vi "Init.vi"(4 "Gyro Full Scale Range":T8, 6 "Accel Full Scale Range":T9, 7 "I2C Channel":u8, 8 "error in (no error)":errorcluster, 9 "Clock Source":u8=1, 10 "Device Address":T10=104 items=["0x68"=104, "0x69"=105], 11 "LINX Resource":T1) -> (0 "error out":errorcluster, 3 "LINX Resource":T1)   [LabVIEW 2011, in "LVH-LINX.lvlib" / "MPU60X0.lvlib"]
doc: "Initializes the MPU-60X0 device setting the clock source and the full ranges for the accelerometer and gyro."
uses:
  <vilib>/LabVIEW Hacker/LINX/Public/Sensors/Accelerometer/MPU60X0/MPU60X0.lvlib
  <vilib>/LabVIEW Hacker/LINX/Public/Sensors/Accelerometer/MPU60X0/DeviceAddresses.ctl
  <vilib>/LabVIEW Hacker/LINX/Public/Sensors/Accelerometer/MPU60X0/AccelFullScaleRanges.ctl
  <vilib>/LabVIEW Hacker/LINX/Public/Sensors/Accelerometer/MPU60X0/GyroFullScaleRanges.ctl
  <vilib>/LabVIEW Hacker/LINX/Private/Type Defs/LINX Ref.ctl
  <vilib>/LabVIEW Hacker/LINX/Private/Type Defs/Platform.ctl
  <vilib>/LabVIEW Hacker/LINX/Private/Type Defs/Interface.ctl
  <vilib>/LabVIEW Hacker/LINX/Private/Device/Type Defs/LINX Device Config.ctl
  <vilib>/LabVIEW Hacker/LINX/Private/Device/Type Defs/TCP Config.ctl
  <vilib>/LabVIEW Hacker/LINX/Private/Type Defs/Device Family.ctl
  <vilib>/LabVIEW Hacker/LINX/Private/Device/Type Defs/Channels.ctl
  <vilib>/LabVIEW Hacker/LINX/LVH-LINX.lvlib
  <vilib>/LabVIEW Hacker/LINX/Private/Device/Device.lvlib
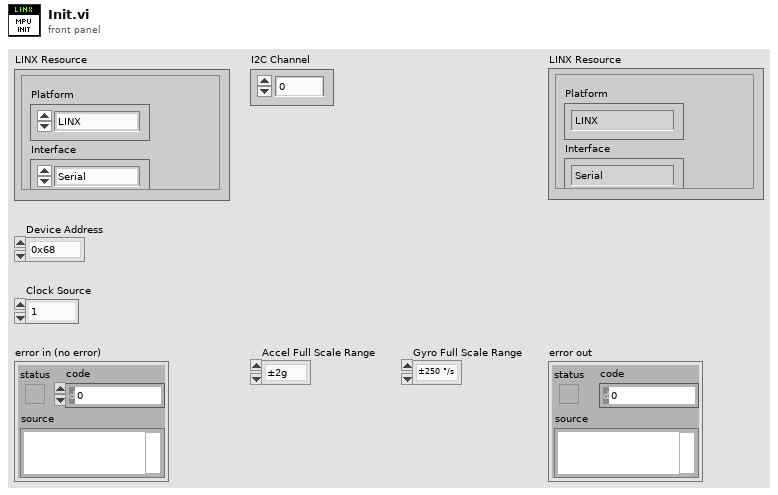
[diagram p1: front panel]
types:
  T1 = typedef "LVH-LINX.lvlib/LINX Ref.ctl" = cluster{"Platform":T2, "Interface":T3, "LINX Device Config":T4}
  T2 = typedef "LVH-LINX.lvlib/Platform.ctl" = enum16{"LINX", "myRIO"}
  T3 = typedef "LVH-LINX.lvlib/Interface.ctl" = enum16{"Serial", "TCP"}
  T4 = typedef "LVH-LINX.lvlib/Device.lvlib/LINX Device Config.ctl" = cluster{"Interface":T3, "COM Port":refnum<visa-resource-name>, "TCP Configuration":T5, "Device Family":T6, "Device ID":u8, "Device Name":string, "TCP Ref":refnum<k5>, "Channels":T7}
  T5 = typedef "LVH-LINX.lvlib/Device.lvlib/TCP Config.ctl" = cluster{"IP Address":string, "Port":u16}
  T6 = typedef "LVH-LINX.lvlib/Device Family.ctl" = enum8{"National Instruments", "Digilent", "Arduino"}
  T7 = typedef "LVH-LINX.lvlib/Channels.ctl" = cluster{"DI Channels":u8[], "DO Channels":u8[], "AI":u8[], "AO":u8[], "PWM":u8[], "QE":u8[], "UART":u8[], "I2C 2":u8[], "SPI":u8[], "CAN":u8[], "AI Ref (V)":dbl, "AO Resolution (Bits)":u8, "AO Ref (V)":dbl}
  T8 = typedef "LVH-LINX.lvlib/MPU60X0.lvlib/GyroFullScaleRanges.ctl" = enum8{"±250 °/s", "±500 °/s", "±1000 °/s", "±2000 °/s"}
  T9 = typedef "LVH-LINX.lvlib/MPU60X0.lvlib/AccelFullScaleRanges.ctl" = enum16{"±2g", "±4g", "±8g", "±16g"}
  T10 = typedef "LVH-LINX.lvlib/MPU60X0.lvlib/DeviceAddresses.ctl" = u8
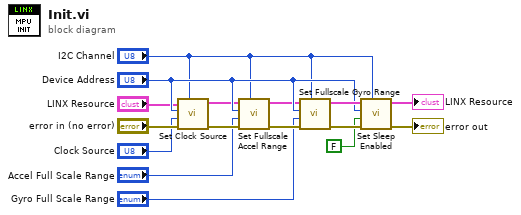
[diagram p0: block diagram]
diagram:
  n1 = call <vilib>:"Set Clock Source.vi"("I2C Channel"="I2C Channel", "error in (no error)"="error in (no error)", "Clock Source"="Clock Source", "Device Address"="Device Address", "LINX Resource"="LINX Resource") -> ("error out"=w13:errorcluster, "LINX Resource"=w4:T1)  [unwired: 5 in]
  n2 = call <vilib>:"Set Fullscale Accel Range.vi"("I2C Channel"="I2C Channel", "error in (no error)"=w13, "Accel Full Scale Range"="Accel Full Scale Range", "Device Address"="Device Address", "LINX Resource"=w4) -> ("error out"=w12:errorcluster, "LINX Resource"=w3:T1)  [unwired: 5 in]
  n3 = call <vilib>:"Set Fullscale Gyro Range.vi"("I2C Channel"="I2C Channel", "error in (no error)"=w12, "Gyro Full Scale Range"="Gyro Full Scale Range", "Device Address"="Device Address", "LINX Resource"=w3) -> ("error out"=w11:errorcluster, "LINX Resource"=w16:T1)  [unwired: 5 in]
  n4 = call <vilib>:"Set Sleep Enabled.vi"("I2C Channel"="I2C Channel", "error in (no error)"=w11, "Sleep?"=FALSE, "Device Address"="Device Address", "LINX Resource"=w16) -> ("error out"=→"error out":errorcluster, "LINX Resource"=→"LINX Resource":T1)  [unwired: 5 in]
